vi "Get Terminal Status Channel.vi"(8 "error in":errorcluster, 11 "terminal":T1 format="%.0x") -> (0 "error out":errorcluster, 2 "status channel":T1 format="%.0x", 3 "terminal out":T1 format="%.0x", 4 "found?":bool)   [LabVIEW 2020, in "AIM MIL-STD-1553 Scripting.lvlib"]
doc: "Returns the <b>status channel</b> for the specified <b>terminal</b>."
uses:
  AIM MIL-STD-1553 Scripting.lvlib
  <vilib>/NI VeriStand/Custom Device API/Custom Device Item Ref.ctl
  Constants.vi
  <vilib>/NI VeriStand/Custom Device Tools/Custom Device Utility Library/NI VeriStand - Search for Item by GUID.vi
  <vilib>/NI VeriStand/Custom Device Tools/Custom Device Utility Library/Custom Device Utility Library.lvlib
  <vilib>/NI VeriStand/Custom Device API/Custom Device API.lvlib
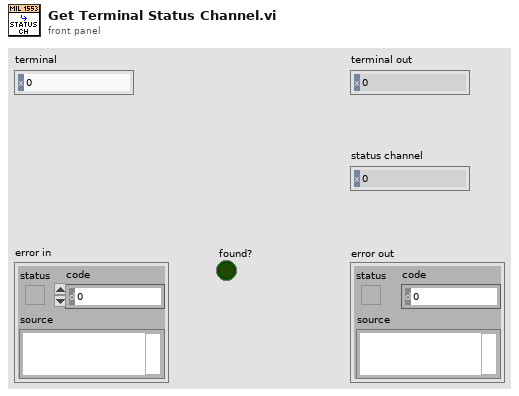
[diagram p1: front panel]
types:
  T1 = typedef "Custom Device API.lvlib/Custom Device Item Ref.ctl" = u64
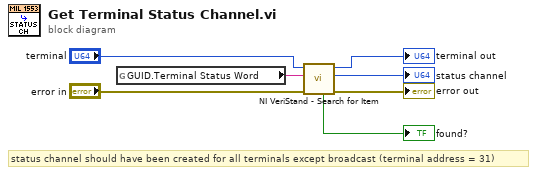
[diagram p0: block diagram]
diagram:
  # "status channel should have been created for all terminals except broadcast (terminal address = 31)"
  n1 = global read "Constants.vi" "GUID.Terminal Status Word"() -> (w6:string)
  n2 = call-poly <vilib>:"NI VeriStand - Search for Item.vi"("error in"="error in", "Item GUID"=w6, "Section Ref in"="terminal") -> ("error out"=→"error out":errorcluster, "Item Ref"=→"status channel":T1, "Section Ref out"=→"terminal out":T1, "Found"=→"found?":bool)  [unwired: 5 in]
